vi "Agorithm.vi"() -> ()   [LabVIEW 2010]
panel:
  in  "Переменные выходные":string[][](table)
  in  "Переменные входные":string[][](table)
  in  "OK Button":bool
  in  "Сообщения Выхлдные":string[][](table)
  in  "Сообщения Входные":string[][](table)
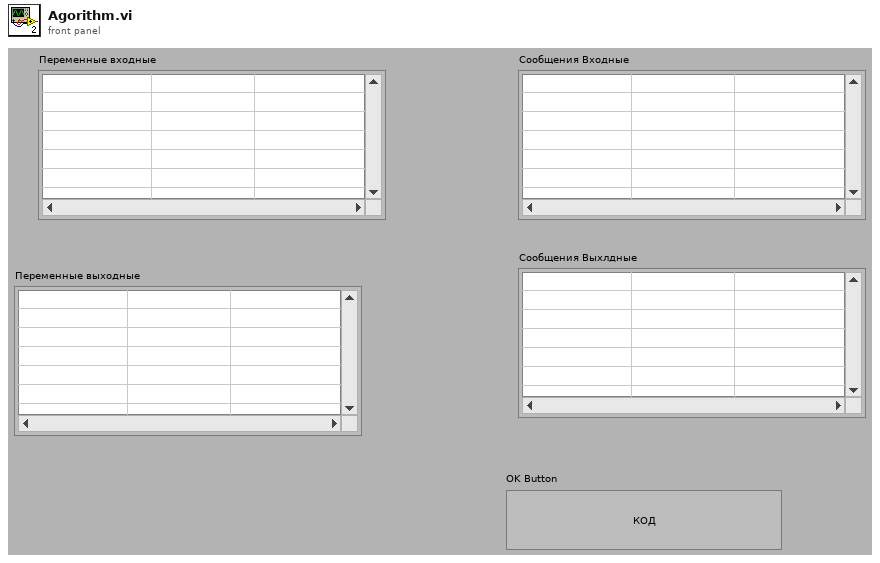
[diagram p1: front panel]
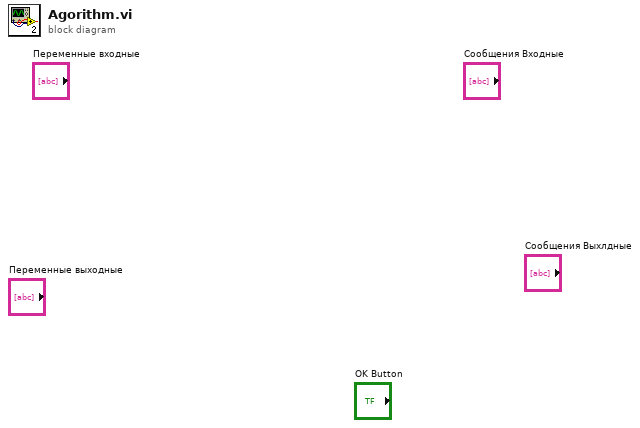
[diagram p0: block diagram]
diagram:
